vi "测量流程.vi"(11 "输入参数":T1) -> ()   [LabVIEW 2016, in "斯坦道总磷总氮.lvlib"]
uses:
  <vilib>/ptbypt/NI_PtbyPt.lvlib
panel:
  out "记录运行时间":timestamp
  out "start":timestamp
  out "重测":bool
  out "x-y":dbl
  out "当前时间":timestamp
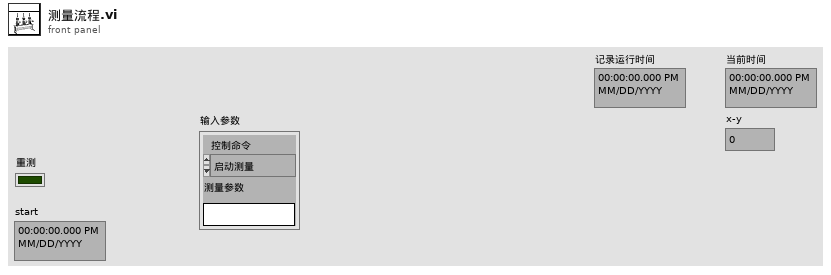
[diagram p1: front panel]
types:
  T1 = typedef "控制命令与参数.ctl" = cluster{"控制命令":enum16{"启动测量", "标样核查", "零点核查", "跨度核查", "空白测试", "平行样测试", "加标回收", "空白校准", "标样校准", "初始化（清洗）", "停止测试", "仪器重启", "校时", "模式设置", "测量间隔设置"}, "测量参数":string}
  T2 = enum16{"启动测量", "标样核查", "零点核查", "跨度核查", "空白测试", "平行样测试", "加标回收", "空白校准", "标样校准", "初始化（清洗）", "停止测试", "仪器重启", "校时", "模式设置", "测量间隔设置"}
  T3 = cluster{"站号":u16, "量程切换":enum32{"H", "L", "AUTO"}, "控制命令":enum16{"启动测量", "标样核查", "零点核查", "跨度核查", "空白测试", "平行样测试", "加标回收", "空白校准", "标样校准", "初始化（清洗）", "停止测试", "仪器重启", "校时", "模式设置", "测量间隔设置"}, "模式设置":enum16{"待机", "连续模式", "周期模式", "定点模式", "受控模式", "手动模式"}, "测量间隔":u16}
  T4 = typedef "操作日志字段定义.ctl" = cluster{"时间":timestamp, "参数":string, "日志信息":string, "流程参数":string}
  T5 = cluster{"时间标识":timestamp, "设备":string, "日志信息":string, "流程参数":string}
  T6 = enum16{"空闲", "水样测试", "标样核查", "零点核查", "跨度核查", "空白测试", "平行样测试", "加标回收", "空白校准", "标样校准", "初始化（清洗）"}
  T7 = cluster{"系统时间":timestamp, "工作状态":u16, "测量模式":enum16{"待机", "连续模式", "周期模式", "定点模式", "受控模式", "手动模式"}, "告警代码":u16, "故障代码":u16, "日志代码":u16, "软件版本":u16, "F0":sgl, "F1":sgl, "F2":sgl, "F3":sgl, "T":sgl, "H":sgl, "id":u16, "flowid":u16, "量程":u16, "总磷控温温度1":sgl, "营养盐控温温度2":sgl, "ADC":sgl, "结果值":sgl, "运行时间":u16, "步骤详情":string, "步骤流程":string}
  T8 = cluster{"水样测试量程模式":enum16{"H", "L", "AUTO"}, "空白核查量程模式":enum16{"H", "L", "AUTO"}, "跨度核查量程模式":enum16{"H", "L", "AUTO"}, "加标回收量程模式":enum16{"H", "L", "AUTO"}, "标样核查量程模式":enum16{"H", "L", "AUTO"}}
  T9 = cluster{"因子编码":u32, "单位":u16, "标样参考值":sgl, "水样数据时间":timestamp, "水样实测值":sgl, "水样数据标识":string, "标样数据时间":timestamp, "标样实测值":sgl, "标样数据标识":string, "空白数据时间":timestamp, "空白实测值":sgl, "空白数据标识":string, "零点核查数据时间":timestamp, "零点核查实测值":sgl, "零点核查数据标识":string, "跨度核查数据时间":timestamp, "跨度核查实测值":sgl, "跨度核查数据标识":string, "加标回收数据时间":timestamp, "加标回收实测值":sgl, "加标回收数据标识":string, "平行样数据时间":timestamp, "平行样实测值":sgl, "平行样数据标识":string, "F0":sgl, "F1":sgl, "F2":sgl, "F3":sgl, "F4":sgl, "F5":sgl, "F6":sgl, "F7":sgl, "温度":sgl, "湿度":sgl, "X值":sgl, "fidrange":u16, "X1值":sgl}[]
  T10 = cluster{"因子编码":u32, "单位":u16, "标样参考值":sgl, "水样数据时间":timestamp, "水样实测值":sgl, "水样数据标识":string, "标样数据时间":timestamp, "标样实测值":sgl, "标样数据标识":string, "空白数据时间":timestamp, "空白实测值":sgl, "空白数据标识":string, "零点核查数据时间":timestamp, "零点核查实测值":sgl, "零点核查数据标识":string, "跨度核查数据时间":timestamp, "跨度核查实测值":sgl, "跨度核查数据标识":string, "加标回收数据时间":timestamp, "加标回收实测值":sgl, "加标回收数据标识":string, "平行样数据时间":timestamp, "平行样实测值":sgl, "平行样数据标识":string, "F0":sgl, "F1":sgl, "F2":sgl, "F3":sgl, "F4":sgl, "F5":sgl, "F6":sgl, "F7":sgl, "温度":sgl, "湿度":sgl, "X值":sgl, "fidrange":u16, "X1值":sgl}
  T11 = cluster{"总磷跨度值":dbl, "总磷零点标准液浓度":dbl, "总磷跨度标准液浓度":dbl, "总磷标准液标准浓度":dbl, "总氮跨度值":dbl, "总氮零点标准液浓度":dbl, "总氮跨度标准液浓度":dbl, "总氮标准液标准浓度":dbl, "COD跨度值":dbl, "COD零点标准液浓度":dbl, "COD跨度标准液浓度":dbl, "COD标准液标准浓度":dbl, "氨氮跨度值":dbl, "氨氮零点标准液浓度":dbl, "氨氮跨度标准液浓度":dbl, "氨氮标准液标准浓度":dbl, "磷酸盐跨度值":dbl, "磷酸盐零点标准液浓度":dbl, "磷酸盐跨度标准液浓度":dbl, "磷酸盐标准液标准浓度":dbl, "硝氮跨度值":dbl, "硝氮零点标准液浓度":dbl, "硝氮跨度标准液浓度":dbl, "硝氮标准液标准浓度":dbl, "亚硝氮跨度值":dbl, "亚硝氮零点标准液浓度":dbl, "亚硝氮跨度标准液浓度":dbl, "亚硝氮标准液标准浓度":dbl, "硫化物跨度值":dbl, "硫化物零点标准液浓度":dbl, "硫化物跨度标准液浓度":dbl, "硫化物标准液标准浓度":dbl, "硅酸盐跨度值":dbl, "硅酸盐零点标准液浓度":dbl, "硅酸盐跨度标准液浓度":dbl, "硅酸盐标准液标准浓度":dbl, "总磷零点标准液偏差":dbl, "总磷跨度标准液偏差":dbl, "总磷标准液标准偏差":dbl, "总氮零点标准液偏差":dbl, "总氮跨度标准液偏差":dbl, "总氮标准液标准偏差":dbl, "COD零点标准液偏差":dbl, "COD跨度标准液偏差":dbl, "COD标准液标准偏差":dbl, "氨氮零点标准液偏差":dbl, "氨氮跨度标准液偏差":dbl, "氨氮标准液标准偏差":dbl, "磷酸盐零点标准液偏差":dbl, "磷酸盐跨度标准液偏差":dbl, "磷酸盐标准液标准偏差":dbl, "硝氮零点标准液偏差":dbl, "硝氮跨度标准液偏差":dbl, "硝氮标准液标准偏差":dbl, "亚硝氮零点标准液偏差":dbl, "亚硝氮跨度标准液偏差":dbl, "亚硝氮标准液标准偏差":dbl, "硫化物零点标准液偏差":dbl, "硫化物跨度标准液偏差":dbl, "硫化物标准液标准偏差":dbl, "硅酸盐零点标准液偏差":dbl, "硅酸盐跨度标准液偏差":dbl, "硅酸盐标准液标准偏差":dbl, "氟化物跨度值":dbl, "氟化物零点标准液浓度":dbl, "氟化物跨度标准液浓度":dbl, "氟化物标准液标准浓度":dbl, "氟化物零点标准液偏差":dbl, "氟化物跨度标准液偏差":dbl, "氟化物标准液标准偏差":dbl, "CODMn跨度值":dbl, "CODMn零点标准液浓度":dbl, "CODMn跨度标准液浓度":dbl, "CODMn标准液标准浓度":dbl, "CODMn零点标准液偏差":dbl, "CODMn跨度标准液偏差":dbl, "CODMn标准液标准偏差":dbl}
  T12 = typedef "LVDateTimeRec.ctl" = cluster{"秒数的小数部分":dbl, "秒":i32, "分":i32, "时":i32, "日":i32, "月":i32, "年":i32, "天数（周）":i32, "天数（年）":i32, "DST":i32}
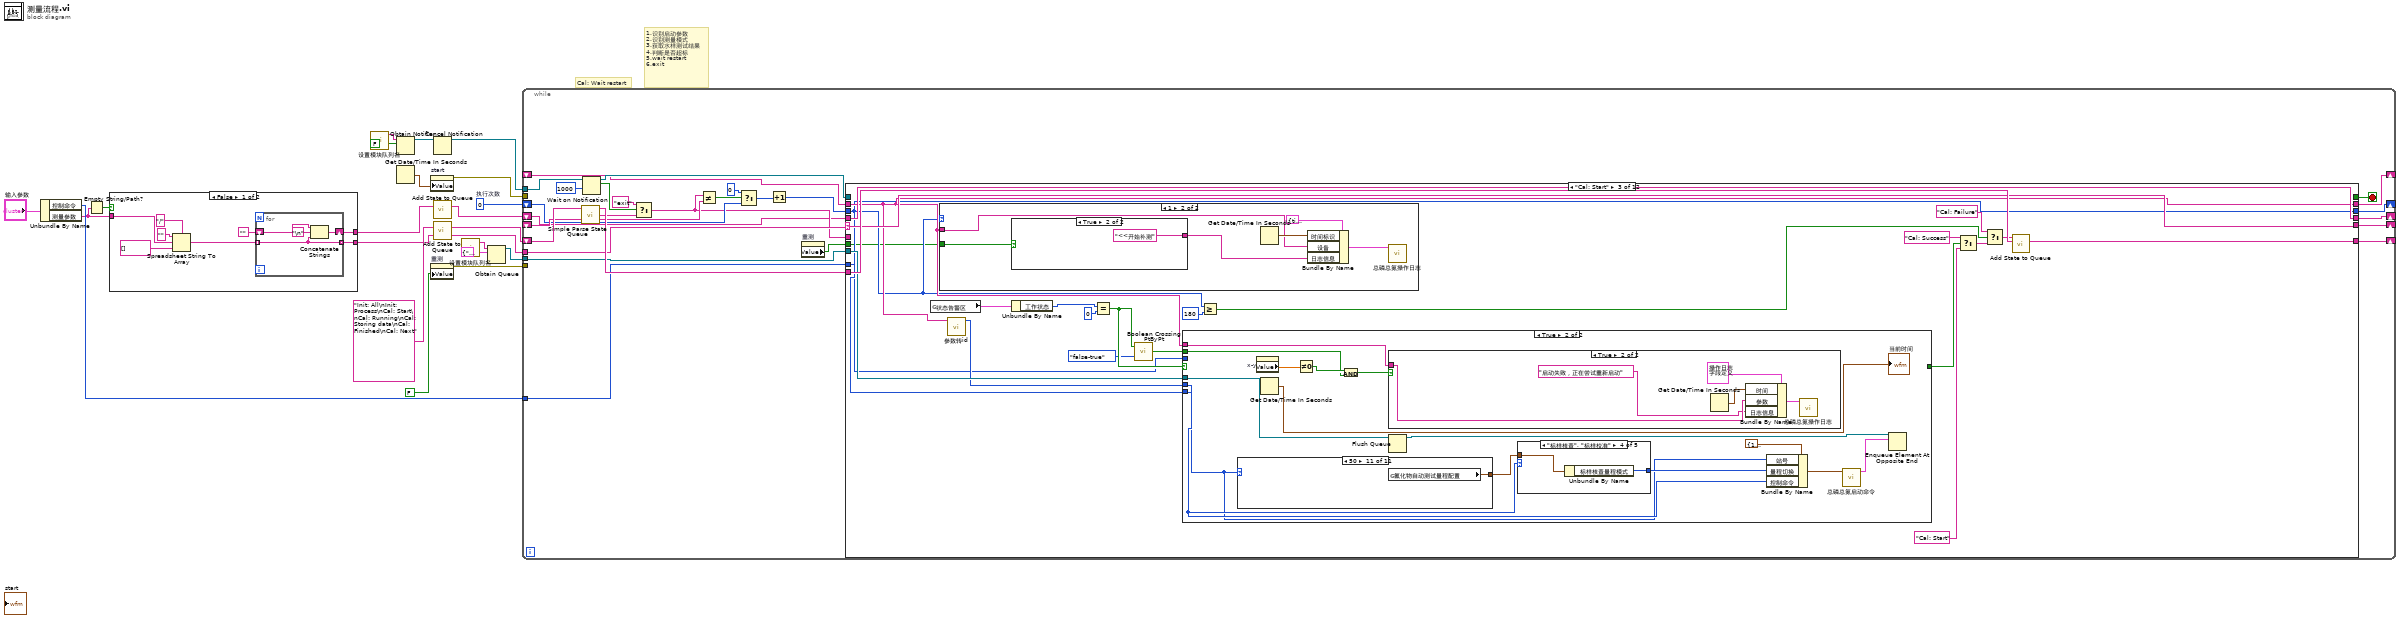
[diagram p0: block diagram]
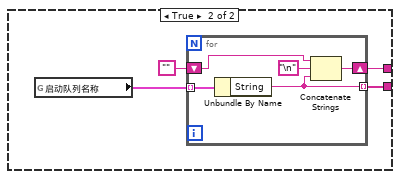
[diagram p2: hidden frame]
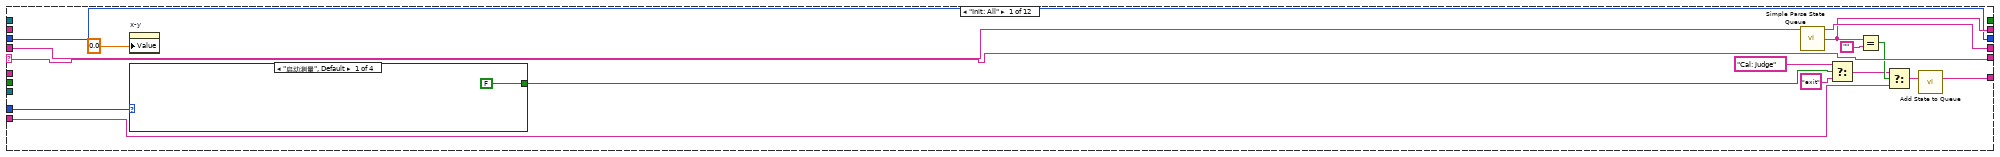
[diagram p3: hidden frame]
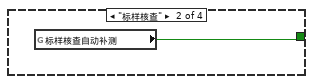
[diagram p4: hidden frame]
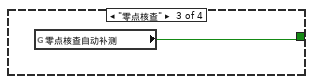
[diagram p5: hidden frame]
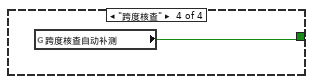
[diagram p6: hidden frame]
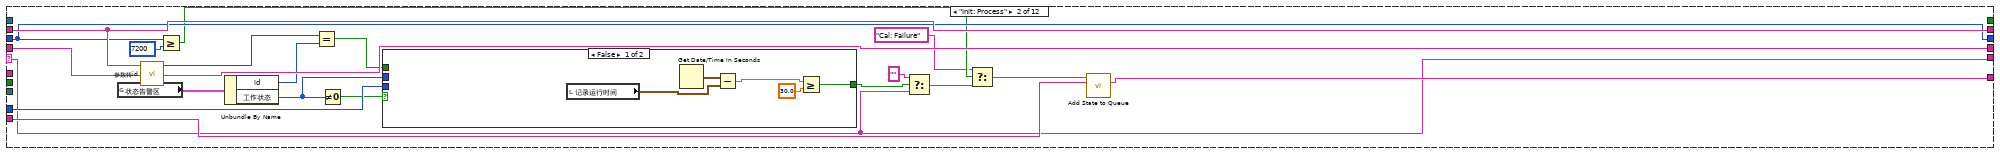
[diagram p7: hidden frame]
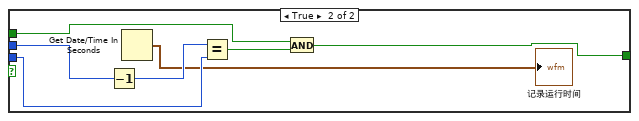
[diagram p8: hidden frame]
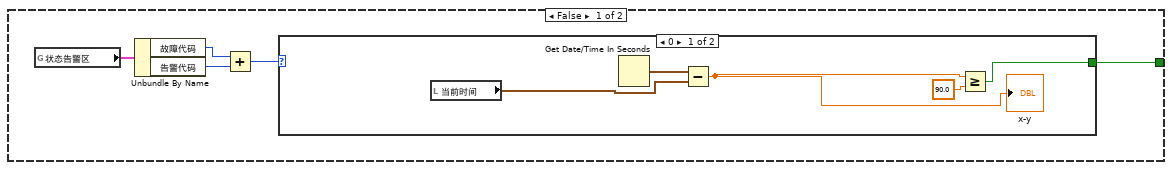
[diagram p9: hidden frame]
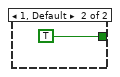
[diagram p10: hidden frame]
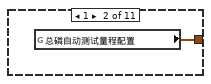
[diagram p13: hidden frame]
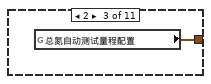
[diagram p14: hidden frame]
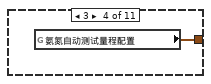
[diagram p15: hidden frame]
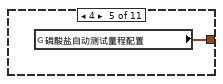
[diagram p16: hidden frame]
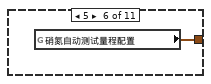
[diagram p17: hidden frame]
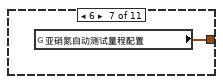
[diagram p18: hidden frame]
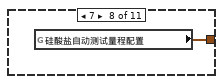
[diagram p19: hidden frame]
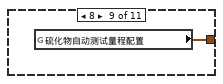
[diagram p20: hidden frame]
diagram:
  w15 = 0  # 执行次数
  # "Cal: Wait restart"
  # "1.识别启动参数\n2.识别测量模式\n3.获取水样测试结果\n4.判断是否超标\n5.wait restart\n6.exit"
  n1 = Unbundle By Name("输入参数") -> ("控制命令"=w3:T2, "测量参数"=w1:string)
  n2 = Empty String/Path?(string/path=w1) -> (empty?=w2:bool)
  n3 = case shown="False" w2 {
    tunnel: [w23 w36] -> w10
    tunnel: [w22 w34] -> w5
    tunnel: w1 -> [w24 _]
    frame False {
      n4 = Spreadsheet String To Array(delimiter (Tab)="/" ("分隔符(Tab)"), format string="" ("格式字符串"), spreadsheet string=w24, array type (2D Dbl)=string[] []) -> (array=w25:string[])
      n5 = for {
        shift-right: [w32] -> w23
        shift-left: "" -> [w33]
        tunnel: w25 -> [w30] mode=indexing
        tunnel: [w30] -> w22 mode=indexing
        n6 = Concatenate Strings(w33, "\n", w30) -> (w32:string)
      }
    }
    frame True {
      n7 = global read "model config var.vi" "启动队列名称"() -> (w35:cluster{"String":string, "Value":u16}[])
      n8 = for {
        shift-right: [w41] -> w36
        shift-left: "" -> [w42]
        tunnel: w35 -> [w40] mode=indexing
        tunnel: [w38] -> w34 mode=indexing
        n9 = Unbundle By Name(w40) -> ("String"=w38:string)
        n10 = Concatenate Strings(w42, "\n", w38) -> (w41:string)
      }
    }
  }
  n11 = call "设置模块队列名.vi"() -> ("Msg"=w13:string)  [unwired: 5 in]
  n12 = Obtain Notifier(name (unnamed)=w13, notification data type=FALSE) -> (notifier out=w20:refnum<notifier>)  [unwired: 2 in, 2 out]
  n13 = Get Date/Time In Seconds() -> (seconds since 1Jan1904=w6:timestamp)
  n14 = property on="start" class="AbsTime (strict)"("Value"=w6) -> (error out=w7:errorcluster)  [unwired: 2 in, 1 out]
  n15 = property on="重测" class="Bool (strict)"("Value"=FALSE ("重测")) -> (error out=w8:errorcluster)  [unwired: 2 in, 1 out]
  n16 = Cancel Notification(0:w20) -> (8:w11:refnum<notifier>)  [unwired: 1 in, 2 out]
  n17 = call "Add State to Queue.vi"("State(s) In (\"\")"=w10) -> ("States Out"=w14:string)  [unwired: 14 in]
  n18 = call "Add State to Queue.vi"("State(s) In (\"\")"="Init: All\nInit: Process\nCal: Start\nCal: Running\nCal: Storing data\nCal: Finished\nCal: Next" ("State(s) In (\"\")")) -> ("States Out"=w18:string)  [unwired: 14 in]
  n19 = call "设置模块队列名.vi"() -> ("Msg"=w12:string)  [unwired: 5 in]
  n20 = Obtain Queue(name (unnamed)=w12, element data type=cluster{"命令":string, "data":variant} {"命令"="", "data"=variant}) -> (queue out=w16:refnum<queue>)  [unwired: 3 in, 2 out]
  n21 = while {
    tunnel: w16 -> [w67]
    shift-right: [w66] -> _
    shift-left: w18 -> [w69]
    shift-right: [w60] -> _
    shift-left: w15 -> [w63]
    shift-right: [w44] -> _
    shift-left: _ -> [w65]
    tunnel: w3 -> [w58]
    shift-right: [w56] -> _
    shift-left: w14 -> [w47]
    shift-right: [w45] -> _
    shift-left: _ -> [w46]
    tunnel: w11 -> [w54]
    tunnel: w8 -> [_]
    tunnel: w7 -> [_]
    tunnel: w5 -> [w43]
    stop <- w57 stop-if-true
    n22 = call "Simple Parse State Queue.vi"("State Queue"=w69) -> ("Remain States"=w68:string, "Next State"=w51:string)  [unwired: 13 in]
    n23 = Wait on Notification(notifier=w54, timeout in ms (-1)=1000 ("超时毫秒(-1)")) -> (notifier out=w49:refnum<notifier>, notification=w53:bool)  [unwired: 2 in, 2 out]
    n24 = Select(t="exit", s=w53, f=w51) -> (s? t:f=w50:string)
    n25 = Not Equal?(x=w50, y=w65) -> (x != y?=w64:bool)
    n26 = Select(t=0, s=w64, f=w63) -> (s? t:f=w61:i32)
    n27 = Increment(x=w61) -> (x+1=w59:i32)
    n28 = property on="重测" class="Bool (strict)"() -> ("Value"=w48:bool)  [unwired: 2 in, 2 out]
    n29 = case shown="\"Cal: Start\"" w50 {
      selector: w50 -> [w84 w98 w143 w208 w223 w229 w243 w260 w277 w290 w454 w475]
      tunnel: w68 -> [w81 w108 w145 w210 _ w240 w248 w262 w274 _ _ w476]
      tunnel: w67 -> [_ _ w141 _ _ _ _ _ _ _ _ w472]
      tunnel: [w85 w109 w144 w209 w224 w239 w247 w261 w273 w278 w462 w476] -> w66
      tunnel: [w84 w98 w143 w208 w223 w229 w243 w260 w277 w290 w454 w475] -> w44
      tunnel: [w75 w97 w123 w207 w222 w232 w246 w258 w272 w291 w465 w474] -> w60
      tunnel: w59 -> [w75 w97 w123 w207 w222 w232 w246 w258 w272 w291 w465 w474]
      tunnel: w58 -> [w74 w102 w140 _ _ _ _ _ _ w289 _ _]
      tunnel: [_ _ _ _ _ _ _ _ _ _ _ TRUE] -> w57
      tunnel: w47 -> [w79 w107 w131 w206 w216 w226 w250 w259 w276 w284 w464 w473]
      tunnel: [w76 w105 w125 w205 w215 w225 w249 w257 w275 w286 w463 w470] -> w45
      tunnel: [w78 w107 w131 w206 w216 w226 w250 w259 w276 w283 w464 w473] -> w56
      tunnel: w46 -> [_ w105 w125 w205 w215 w225 w249 w257 w275 w286 w463 w470]
      tunnel: w49 -> [_ _ _ _ _ _ _ _ _ _ _ w471]
      tunnel: w48 -> [_ _ w122 _ _ _ _ w256 _ w288 _ _]
      tunnel: w43 -> [_ _ _ _ _ _ _ _ _ w285 _ _]
      frame "Init: All" {
        n30 = property on="x-y" class="DigNum (strict)"("Value"=0.0 ("x-y")) -> ()  [unwired: 2 in, 2 out]
        n31 = case shown="\"启动测量\", Default" w74 {
          tunnel: [FALSE ("跨度核查自动补测") w87 w88 w89] -> w73
          frame "启动测量", Default {
          }
          frame "标样核查" {
            n32 = global read "总磷总氮断电保存全局变量.vi" "标样核查自动补测"() -> (w87:bool)
          }
          frame "零点核查" {
            n33 = global read "总磷总氮断电保存全局变量.vi" "零点核查自动补测"() -> (w88:bool)
          }
          frame "跨度核查" {
            n34 = global read "总磷总氮断电保存全局变量.vi" "跨度核查自动补测"() -> (w89:bool)
          }
        }
        n35 = call "Simple Parse State Queue.vi"("State Queue"=w79) -> ("Remain States"=w78:string, "Next State"=w76:string)  [unwired: 13 in]
        n36 = Select(t="Cal: Judge", s=w73, f="exit") -> (s? t:f=w70:string)
        n37 = Equal?(x=w76, y="") -> (x = y?=w77:bool)
        n38 = Select(t=w70, s=w77, f=w81) -> (s? t:f=w80:string)
        n39 = call "Add State to Queue.vi"("State(s) In (\"\")"=w80) -> ("States Out"=w85:string)  [unwired: 14 in]
      }
      frame "Init: Process" {
        n40 = global read "VAR总磷总氮全局变量.vi" "状态告警区"() -> (w106:T7)
        n41 = call "参数转id.vi"("table"=w105) -> ("id"=w103:u16)  [unwired: 10 in]
        n42 = Greater Or Equal?(x=w97, y=7200) -> (x >= y?=w95:bool)
        n43 = Unbundle By Name(w106) -> ("id"=w104:u16, "工作状态"=w100:u16)
        n44 = Equal?(x=w103, y=w104) -> (x = y?=w91:bool)
        n45 = Not Equal To 0?(x=w100) -> (x != 0?=w101:bool)
        n46 = case shown="False" w101 {
          tunnel: w100 -> [_ w121]
          tunnel: w102 -> [_ w119]
          tunnel: [w110 w116] -> w90
          tunnel: w91 -> [_ w117]
          frame False {
            n47 = local read "记录运行时间"() -> (w114:timestamp)
            n48 = Get Date/Time In Seconds() -> (seconds since 1Jan1904=w113:timestamp)
            n49 = Subtract(x=w113, y=w114) -> (x-y=w112:dbl)
            n50 = Greater Or Equal?(x=w112, y=30.0) -> (x >= y?=w110:bool)
          }
          frame True {
            n51 = Decrement(x=w121) -> (x-1=w120:u16)
            n52 = Get Date/Time In Seconds() -> (seconds since 1Jan1904=→"记录运行时间":timestamp)
            n53 = Equal?(x=w120, y=w119) -> (x = y?=w118:bool)
            n54 = And(x=w117, y=w118) -> (x .and. y?=w116:bool)
          }
        }
        n55 = Select(t="", s=w90, f=w98) -> (s? t:f=w93:string)
        n56 = Select(t="Cal: Failure", s=w95, f=w93) -> (s? t:f=w92:string)
        n57 = call "Add State to Queue.vi"("State(s) In Front (\"\")"=w92, "State(s) In (\"\")"=w108) -> ("States Out"=w109:string)  [unwired: 13 in]
      }
      frame "Cal: Start" {
        n58 = global read "VAR总磷总氮全局变量.vi" "状态告警区"() -> (w142:T7)
        n59 = case shown="1" w123 {
          tunnel: w125 -> [_ w198]
          tunnel: w122 -> [_ w197]
          frame 0, Default {
          }
          frame 1 {
            n60 = case shown="True" w197 {
              tunnel: ["<<开始测量" ("日志信息") "<<开始补测" ("日志信息")] -> w199
              frame False {
              }
              frame True {
              }
            }
            n61 = Get Date/Time In Seconds() -> (seconds since 1Jan1904=w202:timestamp)
            n62 = Bundle By Name(cluster=T5 {"时间标识"=timestamp(0 s since 1904-01-01), "设备"="", "日志信息"="", "流程参数"=""} ("data in"), "时间标识"=w202, "设备"=w198, "日志信息"=w199) -> (w201:T5)
            n63 = call "总磷总氮操作日志.vi"("data in"=w201) -> ()  [unwired: 10 in, 1 out]
          }
        }
        n64 = call "参数转id.vi"("table"=w125) -> ("id"=w124:u16)  [unwired: 10 in]
        n65 = Unbundle By Name(w142) -> ("工作状态"=w130:u16)
        n66 = Equal?(x=w130, y=u16 0) -> (x = y?=w128:bool)
        n67 = call <vilib>:"Boolean Crossing PtByPt.vi"("direction"=enum16{"either", "false-true", "true-false"}."false-true", "input"=w128) -> ("crossing"=w126:bool)  [unwired: 1 in]
        n68 = case shown="True" w128 {
          tunnel: w140 -> [_ w167]
          tunnel: w141 -> [_ w170]
          tunnel: [w150 _] -> w135
          tunnel: w124 -> [_ w165]
          tunnel: w123 -> [_ _]
          tunnel: w125 -> [_ w159]
          tunnel: w126 -> [_ w157]
          frame False {
            n69 = global read "VAR总磷总氮全局变量.vi" "状态告警区"() -> (w149:T7)
            n70 = Unbundle By Name(w149) -> ("故障代码"=w147:u16, "告警代码"=w148:u16)
            n71 = Add(x=w147, y=w148) -> (x+y=w146:u16)
            n72 = case shown="0" w146 {
              tunnel: [w151 TRUE] -> w150
              frame 0 {
                n73 = local read "当前时间"() -> (w155:timestamp)
                n74 = Get Date/Time In Seconds() -> (seconds since 1Jan1904=w154:timestamp)
                n75 = Subtract(x=w154, y=w155) -> (x-y=w153:dbl)
                "x-y" <- w153
                n76 = Greater Or Equal?(x=w153, y=90.0) -> (x >= y?=w151:bool)
              }
              frame 1, Default {
              }
            }
          }
          frame True {
            n77 = case shown="50" w165 {
              tunnel: [_ w177 w178 w179 w180 w181 w182 w183 w184 w185 w186] -> w166
              frame 0, Default {
              }
              frame 1 {
                n78 = global read "总磷总氮断电保存全局变量.vi" "总磷自动测试量程配置"() -> (w177:T8)
              }
              frame 2 {
                n79 = global read "总磷总氮断电保存全局变量.vi" "总氮自动测试量程配置"() -> (w178:T8)
              }
              frame 3 {
                n80 = global read "总磷总氮断电保存全局变量.vi" "氨氮自动测试量程配置"() -> (w179:T8)
              }
              frame 4 {
                n81 = global read "总磷总氮断电保存全局变量.vi" "磷酸盐自动测试量程配置"() -> (w180:T8)
              }
              frame 5 {
                n82 = global read "总磷总氮断电保存全局变量.vi" "硝氮自动测试量程配置"() -> (w181:T8)
              }
              frame 6 {
                n83 = global read "总磷总氮断电保存全局变量.vi" "亚硝氮自动测试量程配置"() -> (w182:T8)
              }
              frame 7 {
                n84 = global read "总磷总氮断电保存全局变量.vi" "硅酸盐自动测试量程配置"() -> (w183:T8)
              }
              frame 8 {
                n85 = global read "总磷总氮断电保存全局变量.vi" "硫化物自动测试量程配置"() -> (w184:T8)
              }
              frame 22 {
                n86 = global read "总磷总氮断电保存全局变量.vi" "COD自动测试量程配置"() -> (w185:T8)
              }
              frame 50 {
                n87 = global read "总磷总氮断电保存全局变量.vi" "氟化物自动测试量程配置"() -> (w186:T8)
              }
            }
            n88 = property on="x-y" class="DigNum (strict)"() -> ("Value"=w161:dbl)  [unwired: 2 in, 2 out]
            n89 = Get Date/Time In Seconds() -> (seconds since 1Jan1904=→"当前时间":timestamp)
            n90 = Not Equal To 0?(x=w161) -> (x != 0?=w160:bool)
            n91 = And(x=w160, y=w157) -> (x .and. y?=w158:bool)
            n92 = case shown="True" w158 {
              tunnel: w159 -> [_ w176]
              frame False {
              }
              frame True {
                n93 = Get Date/Time In Seconds() -> (seconds since 1Jan1904=w175:timestamp)
                n94 = Bundle By Name(cluster=T4 {"时间"=timestamp(0 s since 1904-01-01), "参数"="", "日志信息"="", "流程参数"=""} ("data in"), "时间"=w175, "参数"=w176, "日志信息"="启动失败，正在尝试重新启动" ("报警信息")) -> (w172:T4)
                n95 = call "总磷总氮操作日志.vi"("data in"=w172) -> ()  [unwired: 10 in, 1 out]
              }
            }
            n96 = Flush Queue(queue=w170) -> (queue out=w163:refnum<queue>)  [unwired: 1 in, 2 out]
            n97 = case shown="\"标样核查\", \"标样校准\"" w167 {
              tunnel: w166 -> [w188 w190 w192 w194 w196]
              tunnel: [w187 w189 w191 w193 w195] -> w171
              frame "启动测量", Default {
                n98 = Unbundle By Name(w188) -> ("水样测试量程模式"=w187:enum16{"H", "L", "AUTO"})
              }
              frame "零点核查", "空白测试", "空白校准" {
                n99 = Unbundle By Name(w190) -> ("空白核查量程模式"=w189:enum16{"H", "L", "AUTO"})
              }
              frame "跨度核查" {
                n100 = Unbundle By Name(w192) -> ("跨度核查量程模式"=w191:enum16{"H", "L", "AUTO"})
              }
              frame "标样核查", "标样校准" {
                n101 = Unbundle By Name(w194) -> ("标样核查量程模式"=w193:enum16{"H", "L", "AUTO"})
              }
              frame "加标回收" {
                n102 = Unbundle By Name(w196) -> ("加标回收量程模式"=w195:enum16{"H", "L", "AUTO"})
              }
            }
            n103 = Bundle By Name(cluster=T3 {"站号"=1, "量程切换"=enum."AUTO", "控制命令"=enum."启动测量", "模式设置"=enum."待机", "测量间隔"=0} ("参数"), "站号"=w165, "量程切换"=w171, "控制命令"=w167) -> (w168:T3)
            n104 = call "总磷总氮启动命令.vi"("参数"=w168) -> ("启动命令"=w164:cluster{"命令":string, "data":variant})  [unwired: 10 in]
            n105 = Enqueue Element At Opposite End(queue=w163, element=w164) -> ()  [unwired: 2 in, 3 out]
          }
        }
        n106 = Greater Or Equal?(x=w123, y=180) -> (x >= y?=w138:bool)
        n107 = Select(t="Cal: Success" ("State(s) In (\"\")"), s=w135, f="Cal: Start" ("State(s) In (\"\")")) -> (s? t:f=w133:string)
        n108 = Select(t="Cal: Failure" ("State(s) In (\"\")"), s=w138, f=w133) -> (s? t:f=w136:string)
        n109 = call "Add State to Queue.vi"("State(s) In Front (\"\")"=w136, "State(s) In (\"\")"=w145) -> ("States Out"=w144:string)  [unwired: 13 in]
      }
      frame "Cal: Success" {
        n110 = Get Date/Time In Seconds() -> (seconds since 1Jan1904=w213:timestamp)
        n111 = Bundle By Name(cluster=T5 {"时间标识"=timestamp(0 s since 1904-01-01), "设备"="", "日志信息"="", "流程参数"=""} ("data in"), "时间标识"=w213, "设备"=w205, "日志信息"="启动成功") -> (w212:T5)
        n112 = call "总磷总氮操作日志.vi"("data in"=w212) -> ()  [unwired: 10 in, 1 out]
        n113 = call "Add State to Queue.vi"("State(s) In (\"\")"=w210) -> ("States Out"=w209:string)  [unwired: 14 in]
      }
      frame "Cal: Failure" {
        n114 = Get Date/Time In Seconds() -> (seconds since 1Jan1904=w220:timestamp)
        n115 = Bundle By Name(cluster=T5 {"时间标识"=timestamp(0 s since 1904-01-01), "设备"="", "日志信息"="", "流程参数"=""} ("data in"), "时间标识"=w220, "设备"=w215, "日志信息"="启动失败") -> (w219:T5)
        n116 = call "总磷总氮操作日志.vi"("data in"=w219) -> ()  [unwired: 10 in, 1 out]
        n117 = call "Add State to Queue.vi"("State(s) In (\"\")"="exit" ("State(s) In (\"\")")) -> ("States Out"=w224:string)  [unwired: 14 in]
      }
      frame "Cal: Running" {
        n118 = global read "VAR总磷总氮全局变量.vi" "状态告警区"() -> (w236:T7)
        n119 = Less Or Equal?(x=w232, y=7200) -> (x <= y?=w230:bool)
        n120 = Unbundle By Name(w236) -> ("工作状态"=w237:u16)
        n121 = Select(t=w229, s=w230, f="exit") -> (s? t:f=w228:string)
        n122 = Equal?(x=w237, y=T6."空闲") -> (x = y?=w235:bool)
        n123 = Select(t="", s=w235, f=w228) -> (s? t:f=w233:string)
        n124 = call "Add State to Queue.vi"("State(s) In Front (\"\")"=w233, "State(s) In (\"\")"=w240) -> ("States Out"=w239:string)  [unwired: 13 in]
      }
      frame "Cal: Storing data" {
        n125 = case shown="1" w246 {
          tunnel: w249 -> [_ w251]
          frame 0, Default {
          }
          frame 1 {
            n126 = Get Date/Time In Seconds() -> (seconds since 1Jan1904=w255:timestamp)
            n127 = Bundle By Name(cluster=T5 {"时间标识"=timestamp(0 s since 1904-01-01), "设备"="", "日志信息"="", "流程参数"=""} ("data in"), "时间标识"=w255, "设备"=w251, "日志信息"="存储数据") -> (w254:T5)
            n128 = call "总磷总氮操作日志.vi"("data in"=w254) -> ()  [unwired: 10 in, 1 out]
          }
        }
        n129 = Less Or Equal?(x=w246, y=60) -> (x <= y?=w244:bool)
        n130 = Select(t=w243, s=w244, f="") -> (s? t:f=w241:string)
        n131 = call "Add State to Queue.vi"("State(s) In Front (\"\")"=w241, "State(s) In (\"\")"=w248) -> ("States Out"=w247:string)  [unwired: 13 in]
      }
      frame "Cal: Finished" {
        n132 = case shown="1" w258 {
          tunnel: w257 -> [_ w264]
          tunnel: w256 -> [_ w263]
          frame 0, Default {
          }
          frame 1 {
            n133 = case shown="False" w263 {
              tunnel: ["测量结束>>" ("日志信息") "补测结束>>" ("日志信息")] -> w265
              frame False {
              }
              frame True {
              }
            }
            n134 = Get Date/Time In Seconds() -> (seconds since 1Jan1904=w268:timestamp)
            n135 = Bundle By Name(cluster=T5 {"时间标识"=timestamp(0 s since 1904-01-01), "设备"="", "日志信息"="", "流程参数"=""} ("data in"), "时间标识"=w268, "设备"=w264, "日志信息"=w265) -> (w267:T5)
            n136 = call "总磷总氮操作日志.vi"("data in"=w267) -> ()  [unwired: 10 in, 1 out]
          }
        }
        n137 = call "Add State to Queue.vi"("State(s) In (\"\")"=w262) -> ("States Out"=w261:string)  [unwired: 14 in]
      }
      frame "Cal: Next" {
        n138 = call "Add State to Queue.vi"("State(s) In Front (\"\")"="Init: All\nInit: Process\nCal: Start\nCal: Running\nCal: Storing data\nCal: Finished\nCal: Next" ("State(s) In (\"\")"), "State(s) In (\"\")"=w274) -> ("States Out"=w273:string)  [unwired: 13 in]
      }
      frame "Cal: Judge" {
        n139 = Not(x=w288) -> (.not. x?=w287:bool)
        n140 = for {
          tunnel: w289 -> [w298]
          tunnel: w287 -> [w297]
          tunnel: w285 -> [w296] mode=indexing
          shift-right: [w294] -> w283
          shift-left: w284 -> [w295]
          shift-right: [w293] -> w281
          shift-left: FALSE -> [w292]
          n141 = case shown="True" w297 {
            tunnel: w298 -> [_ w312]
            tunnel: w296 -> [_ w305]
            tunnel: w295 -> [_ w304]
            tunnel: ["" ("States Out") w303] -> w294
            tunnel: [FALSE w302] -> w293
            tunnel: w292 -> [_ w301]
            frame False {
              # "继续测试下一个参数/EXIT"
            }
            frame True {
              # "参数测完-判定是否超标"
              n142 = call "参数转id.vi"("table"=w305) -> ("id"=w306:u16)  [unwired: 10 in]
              n143 = call "id参数转换.vi"("id"=w306) -> ("数组资源索引"=w311:i32)  [unwired: 9 in, 1 out]
              n144 = global read "VAR总磷总氮全局变量.vi" "测量数据区数组"() -> (w310:T9)
              n145 = Index Array(array=w310, index=w311) -> (element=w309:T10)
              n146 = case shown="\"跨度核查\"" w312 {
                tunnel: w309 -> [_ w331 w382 w422]
                tunnel: w306 -> [_ w329 w383 w421]
                tunnel: [TRUE w327 w380 w419] -> w308
                tunnel: [_ "标样核查不合格" ("日志信息") "零点核查不合格" ("日志信息") "跨度核查不合格" ("日志信息")] -> w307
                frame "启动测量", Default {
                }
                frame "标样核查" {
                  n147 = Unbundle By Name(w331) -> ("标样实测值"=w324:sgl)
                  n148 = global read "总磷总氮断电保存全局变量.vi" "质控参数设置"() -> (w330:T11)
                  n149 = case shown="5" w329 {
                    tunnel: w330 -> [_ w334 w337 w340 w343 w346 w349 w356 w363 w370 w377]
                    tunnel: [_ w333 w336 w339 w342 w345 w348 w355 w362 w369 w376] -> w326
                    tunnel: [_ w332 w335 w338 w341 w344 w347 w354 w361 w368 w375] -> w325
                    frame Default {
                    }
                    frame 1 {
                      n150 = Unbundle By Name(w334) -> ("总磷标准液标准浓度"=w333:dbl, "总磷标准液标准偏差"=w332:dbl)
                    }
                    frame 2 {
                      n151 = Unbundle By Name(w337) -> ("总氮标准液标准浓度"=w336:dbl, "总氮标准液标准偏差"=w335:dbl)
                    }
                    frame 3 {
                      n152 = Unbundle By Name(w340) -> ("氨氮标准液标准浓度"=w339:dbl, "氨氮标准液标准偏差"=w338:dbl)
                    }
                    frame 4 {
                      n153 = Unbundle By Name(w343) -> ("磷酸盐标准液标准浓度"=w342:dbl, "磷酸盐标准液标准偏差"=w341:dbl)
                    }
                    frame 5 {
                      n154 = Unbundle By Name(w346) -> ("硝氮标准液标准浓度"=w345:dbl, "硝氮标准液标准偏差"=w344:dbl)
                    }
                    frame 6 {
                      n155 = Unbundle By Name(w349) -> ("亚硝氮标准液标准浓度"=w351:dbl, "亚硝氮标准液标准偏差"=w353:dbl)
                      n156 = Multiply(x=w353, y=0.01) -> (x*y=w350:dbl)
                      n157 = Add(x=w351, y=w350) -> (x+y=w348:dbl)
                      n158 = Subtract(x=w351, y=w350) -> (x-y=w347:dbl)
                    }
                    frame 7 {
                      n159 = Unbundle By Name(w356) -> ("硅酸盐标准液标准浓度"=w358:dbl, "硅酸盐标准液标准偏差"=w360:dbl)
                      n160 = Multiply(x=w360, y=0.01) -> (x*y=w357:dbl)
                      n161 = Add(x=w358, y=w357) -> (x+y=w355:dbl)
                      n162 = Subtract(x=w358, y=w357) -> (x-y=w354:dbl)
                    }
                    frame 8 {
                      n163 = Unbundle By Name(w363) -> ("硫化物标准液标准浓度"=w365:dbl, "硫化物标准液标准偏差"=w367:dbl)
                      n164 = Multiply(x=w367, y=0.01) -> (x*y=w364:dbl)
                      n165 = Add(x=w365, y=w364) -> (x+y=w362:dbl)
                      n166 = Subtract(x=w365, y=w364) -> (x-y=w361:dbl)
                    }
                    frame 22 {
                      n167 = Unbundle By Name(w370) -> ("COD标准液标准浓度"=w372:dbl, "COD标准液标准偏差"=w374:dbl)
                      n168 = Multiply(x=w374, y=0.01) -> (x*y=w371:dbl)
                      n169 = Add(x=w372, y=w371) -> (x+y=w369:dbl)
                      n170 = Subtract(x=w372, y=w371) -> (x-y=w368:dbl)
                    }
                    frame 50 {
                      n171 = Unbundle By Name(w377) -> ("氟化物标准液标准浓度"=w376:dbl, "氟化物标准液标准偏差"=w375:dbl)
                    }
                  }
                  n172 = call "相对标准偏差判断.vi"("实测值"=w324, "相对标准偏差"=w325, "标样值"=w326) -> ("合格？"=w327:bool)  [unwired: 8 in]
                }
                frame "零点核查" {
                  n173 = Unbundle By Name(w382) -> ("零点核查实测值"=w378:sgl)
                  n174 = global read "总磷总氮断电保存全局变量.vi" "质控参数设置"() -> (w385:T11)
                  n175 = case shown="3" w383 {
                    tunnel: w385 -> [_ w388 w391 w394 w397 w400 w403 w406 w409 w412 w415]
                    tunnel: [_ w387 w390 w393 w396 w399 w402 w405 w408 w411 w414] -> w384
                    tunnel: [_ w386 w389 w392 w395 w398 w401 w404 w407 w410 w413] -> w379
                    frame Default {
                    }
                    frame 1 {
                      n176 = Unbundle By Name(w388) -> ("总磷零点标准液浓度"=w387:dbl, "总磷零点标准液偏差"=w386:dbl)
                    }
                    frame 2 {
                      n177 = Unbundle By Name(w391) -> ("总氮零点标准液浓度"=w390:dbl, "总氮零点标准液偏差"=w389:dbl)
                    }
                    frame 3 {
                      n178 = Unbundle By Name(w394) -> ("氨氮零点标准液浓度"=w393:dbl, "氨氮零点标准液偏差"=w392:dbl)
                    }
                    frame 4 {
                      n179 = Unbundle By Name(w397) -> ("磷酸盐零点标准液浓度"=w396:dbl, "磷酸盐零点标准液偏差"=w395:dbl)
                    }
                    frame 5 {
                      n180 = Unbundle By Name(w400) -> ("硝氮零点标准液浓度"=w399:dbl, "硝氮零点标准液偏差"=w398:dbl)
                    }
                    frame 6 {
                      n181 = Unbundle By Name(w403) -> ("亚硝氮零点标准液浓度"=w402:dbl, "亚硝氮零点标准液偏差"=w401:dbl)
                    }
                    frame 7 {
                      n182 = Unbundle By Name(w406) -> ("硅酸盐零点标准液浓度"=w405:dbl, "硅酸盐零点标准液偏差"=w404:dbl)
                    }
                    frame 8 {
                      n183 = Unbundle By Name(w409) -> ("硫化物零点标准液浓度"=w408:dbl, "硫化物零点标准液偏差"=w407:dbl)
                    }
                    frame 22 {
                      n184 = Unbundle By Name(w412) -> ("COD零点标准液浓度"=w411:dbl, "COD零点标准液偏差"=w410:dbl)
                    }
                    frame 50 {
                      n185 = Unbundle By Name(w415) -> ("氟化物零点标准液浓度"=w414:dbl, "氟化物零点标准液偏差"=w413:dbl)
                    }
                  }
                  n186 = call "绝对标准偏差判断.vi"("实测值"=w378, "绝对标准偏差"=w379, "标准值"=w384) -> ("合格？"=w380:bool)  [unwired: 8 in]
                }
                frame "跨度核查" {
                  n187 = Unbundle By Name(w422) -> ("跨度核查实测值"=w418:sgl)
                  n188 = global read "总磷总氮断电保存全局变量.vi" "质控参数设置"() -> (w423:T11)
                  n189 = case shown="1" w421 {
                    tunnel: w423 -> [_ w426 w429 w432 w435 w438 w441 w444 w447 w450 w453]
                    tunnel: [_ w425 w428 w431 w434 w437 w440 w443 w446 w449 w452] -> w417
                    tunnel: [_ w424 w427 w430 w433 w436 w439 w442 w445 w448 w451] -> w416
                    frame Default {
                    }
                    frame 1 {
                      n190 = Unbundle By Name(w426) -> ("总磷跨度标准液浓度"=w425:dbl, "总磷跨度标准液偏差"=w424:dbl)
                    }
                    frame 2 {
                      n191 = Unbundle By Name(w429) -> ("总氮跨度标准液浓度"=w428:dbl, "总氮跨度标准液偏差"=w427:dbl)
                    }
                    frame 3 {
                      n192 = Unbundle By Name(w432) -> ("氨氮跨度标准液浓度"=w431:dbl, "氨氮跨度标准液偏差"=w430:dbl)
                    }
                    frame 4 {
                      n193 = Unbundle By Name(w435) -> ("磷酸盐跨度标准液浓度"=w434:dbl, "磷酸盐跨度标准液偏差"=w433:dbl)
                    }
                    frame 5 {
                      n194 = Unbundle By Name(w438) -> ("硝氮跨度标准液浓度"=w437:dbl, "硝氮跨度标准液偏差"=w436:dbl)
                    }
                    frame 6 {
                      n195 = Unbundle By Name(w441) -> ("亚硝氮跨度标准液浓度"=w440:dbl, "亚硝氮跨度标准液偏差"=w439:dbl)
                    }
                    frame 7 {
                      n196 = Unbundle By Name(w444) -> ("硅酸盐跨度标准液浓度"=w443:dbl, "硅酸盐跨度标准液偏差"=w442:dbl)
                    }
                    frame 8 {
                      n197 = Unbundle By Name(w447) -> ("硫化物跨度标准液浓度"=w446:dbl, "硫化物跨度标准液偏差"=w445:dbl)
                    }
                    frame 22 {
                      n198 = Unbundle By Name(w450) -> ("COD跨度标准液浓度"=w449:dbl, "COD跨度标准液偏差"=w448:dbl)
                    }
                    frame 50 {
                      n199 = Unbundle By Name(w453) -> ("氟化物跨度标准液浓度"=w452:dbl, "氟化物跨度标准液偏差"=w451:dbl)
                    }
                  }
                  n200 = call "相对标准偏差判断.vi"("实测值"=w418, "相对标准偏差"=w416, "标样值"=w417) -> ("合格？"=w419:bool)  [unwired: 8 in]
                }
              }
              n201 = case shown="False" w308 {
                tunnel: w305 -> [w314 _]
                tunnel: w307 -> [w317 _]
                tunnel: w304 -> [w316 w322]
                tunnel: [w315 w322] -> w303
                tunnel: [TRUE w321] -> w302
                tunnel: w301 -> [_ w321]
                frame False {
                  n202 = call "Add State to Queue.vi"("State(s) In (\"\")"=w316, "State(s) At Back (\"\")"=w314) -> ("States Out"=w315:string)  [unwired: 13 in]
                  n203 = Get Date/Time In Seconds() -> (seconds since 1Jan1904=w320:timestamp)
                  n204 = Bundle By Name(cluster=T5 {"时间标识"=timestamp(0 s since 1904-01-01), "设备"="", "日志信息"="", "流程参数"=""} ("data in"), "时间标识"=w320, "设备"=w314, "日志信息"=w317) -> (w319:T5)
                  n205 = call "总磷总氮操作日志.vi"("data in"=w319) -> ()  [unwired: 10 in, 1 out]
                }
                frame True {
                }
              }
            }
          }
        }
        n206 = Select(t="Cal: Wait restart" ("State(s) In (\"\")"), s=w281, f="exit" ("State(s) In (\"\")")) -> (s? t:f=w278:string)
      }
      frame "Cal: Wait restart" {
        n207 = local read "start"() -> (w461:timestamp)
        n208 = Get Date/Time In Seconds() -> (seconds since 1Jan1904=w458:timestamp)
        n209 = Seconds To Date/Time(time stamp (now)=w461) -> (date time rec=w460:T12)  [unwired: 1 in]
        n210 = Seconds To Date/Time(time stamp (now)=w458) -> (date time rec=w459:T12)  [unwired: 1 in]
        n211 = Unbundle By Name(w460) -> ("时"=w456:i32)
        n212 = Unbundle By Name(w459) -> ("时"=w457:i32)
        n213 = Not Equal?(x=w456, y=w457) -> (x != y?=w455:bool)
        n214 = case shown="True" w455 {
          tunnel: [w466 "Init: All\nInit: Process\nCal: Start\nCal: Running\nCal: Storing data\nCal: Finished\nCal: Next" ("State(s) In (\"\")")] -> w462
          tunnel: w454 -> [w466 _]
          frame False {
          }
          frame True {
            "重测" <- TRUE ("重测")
          }
        }
      }
      frame "exit", Default {
        n215 = Release Notifier(notifier=w471) -> ()  [unwired: 2 in, 3 out]
        n216 = Release Queue(queue=w472) -> ()  [unwired: 2 in, 3 out]
        n217 = Empty String/Path?(string/path=w470) -> (empty?=w469:bool)
        n218 = case shown="False" w469 {
          tunnel: w470 -> [w478 _]
          frame False {
            n219 = Get Date/Time In Seconds() -> (seconds since 1Jan1904=w482:timestamp)
            n220 = Bundle By Name(cluster=T5 {"时间标识"=timestamp(0 s since 1904-01-01), "设备"="", "日志信息"="", "流程参数"=""} ("data in"), "时间标识"=w482, "设备"=w478, "日志信息"="流程结束>>") -> (w481:T5)
            n221 = call "总磷总氮操作日志.vi"("data in"=w481) -> ()  [unwired: 10 in, 1 out]
          }
          frame True {
          }
        }
      }
    }
  }
